vi "Send Get Table.vi"(6 "timeout in ms (-1)":i32=-1, 7 "Message Priority (Normal)":T1=enum."Normal", 8 "error in (no error)":errorcluster, 11 "Message Enqueuer":refnum<class "Message Enqueuer.lvclass">) -> (0 "error out":errorcluster, 2 "Table":refnum<class "Basic Table.lvclass">, 3 "Message Enqueuer out":refnum<class "Message Enqueuer.lvclass">, 4 "timed out?":bool)   [LabVIEW 2020, in "Panel Form Controller.lvlib" / "Get Table Msg.lvclass"]
doc: "This VI sends the message to an actor."
uses:
  Get Table Msg.lvclass
  <vilib>/ActorFramework/Message Enqueuer/Message Enqueuer.lvclass
  <vilib>/ActorFramework/Message Enqueuer/Message Priority.ctl
  Database OOP/Table Libraries/Basic Table/Basic Table Class/Basic Table.lvclass
  C:/Program Files (x86)/National Instruments/LabVIEW 2020/vi.lib/ActorFramework/Reply Msg/Reply Msg.lvclass
  <vilib>/ActorFramework/Reply Msg/Reply Msg.lvclass/Reply Msg.ctl
  <vilib>/ActorFramework/Message Enqueuer/Message Enqueuer.lvclass/Message Enqueuer.ctl
  <vilib>/ActorFramework/Message Enqueuer/Enqueue.vi
  <vilib>/ActorFramework/Reply Msg/Reply Msg.lvclass
  C:/Program Files (x86)/National Instruments/LabVIEW 2020/vi.lib/ActorFramework/Message/Message.lvclass
  <vilib>/ActorFramework/Message Priority Queue/Priority Enqueue.vi
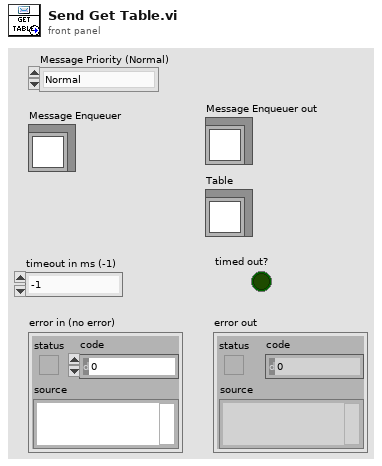
[diagram p1: front panel]
types:
  T1 = typedef "Actor Framework.lvlib/Message Enqueuer.lvclass/Message Priority.ctl" = enum16{"Low", "Normal", "High"}
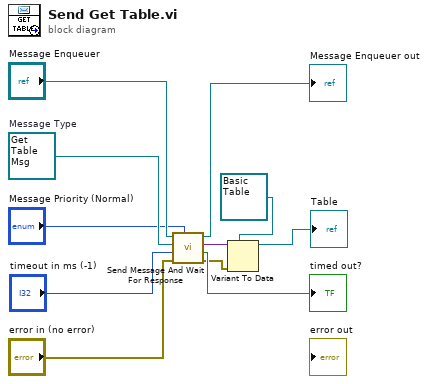
[diagram p0: block diagram]
diagram:
  w9 = refnum<class "Get Table Msg.lvclass"> refnum  # Message Type
  n1 = call <vilib>:"Send Message And Wait For Response.vi"("Message Priority (Normal)"="Message Priority (Normal)", "error in (no error)"="error in (no error)", "timeout in ms (-1)"="timeout in ms (-1)", "Original Message"=w9, "Message Enqueuer in"="Message Enqueuer") -> ("error out"=w3:errorcluster, "timed out?"=→"timed out?":bool, "Reply"=w4:variant, "Message Enqueuer out"=→"Message Enqueuer out":refnum<class "Message Enqueuer.lvclass">)  [unwired: 3 in]
  n2 = Variant To Data(error in=w3, type=refnum<class "Basic Table.lvclass"> refnum ("Table.lvlib:Basic Table.lvclass"), Variant=w4) -> (data=→"Table":refnum<class "Basic Table.lvclass">)  [unwired: 1 out]
